vi "Finish.vi"(8 "error in (no error)":errorcluster, 11 "Demo Mode in":refnum<class "Demo Mode.lvclass">) -> (0 "error out":errorcluster, 3 "Demo Mode out":refnum<class "Demo Mode.lvclass">)   [LabVIEW 2019, in "Joysticks.lvlib" / "Demo Mode.lvclass"]
doc: "Use this method to close the references to the joysticks."
uses:
  Demo Mode.lvclass
  Joysticks.lvclass
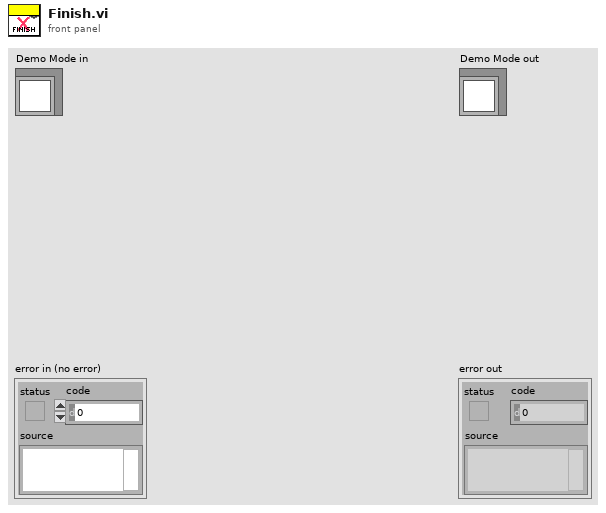
[diagram p1: front panel]
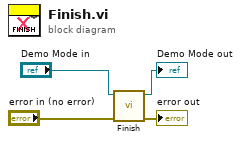
[diagram p0: block diagram]
diagram:
  n1 = call-parent "Finish.vi"("error in (no error)"="error in (no error)", "Joysticks in"="Demo Mode in") -> ("error out"=→"error out":errorcluster, "Joysticks out"=→"Demo Mode out":refnum<class "Demo Mode.lvclass">)  [unwired: 8 in]
